vi "MoveVelocity.vi"(0 "reinitialize? (F)":bool, 1 "PID gains":T1={"proportional gain (Kc)"=0.6, "integral time (Ti, min)"=0.001, "derivative time (Td, min)"=0.0002}, 2 "output range":cluster{"output high":dbl, "output low":dbl}={"output high"=100.0, "output low"=-100.0}, 7 "EncRst":bool, 9 "OBJ":dbl[](array[numeric]), 11 "error in (no error)":errorcluster, 12 "dt (s)":dbl=0.010000000000000002 format="%#_13g") -> (6 "power":dbl[](array[numeric]), 8 "®t­È":dbl[](array[numeric]), 10 "Enc":dbl[](array[numeric]), 15 "error out":errorcluster)   [LabVIEW 2019]
uses:
  <vilib>/addons/control/pid/pid.llb/PID (DBL).vi
  <vilib>/addons/control/pid/NI_PID_pid.lvlib
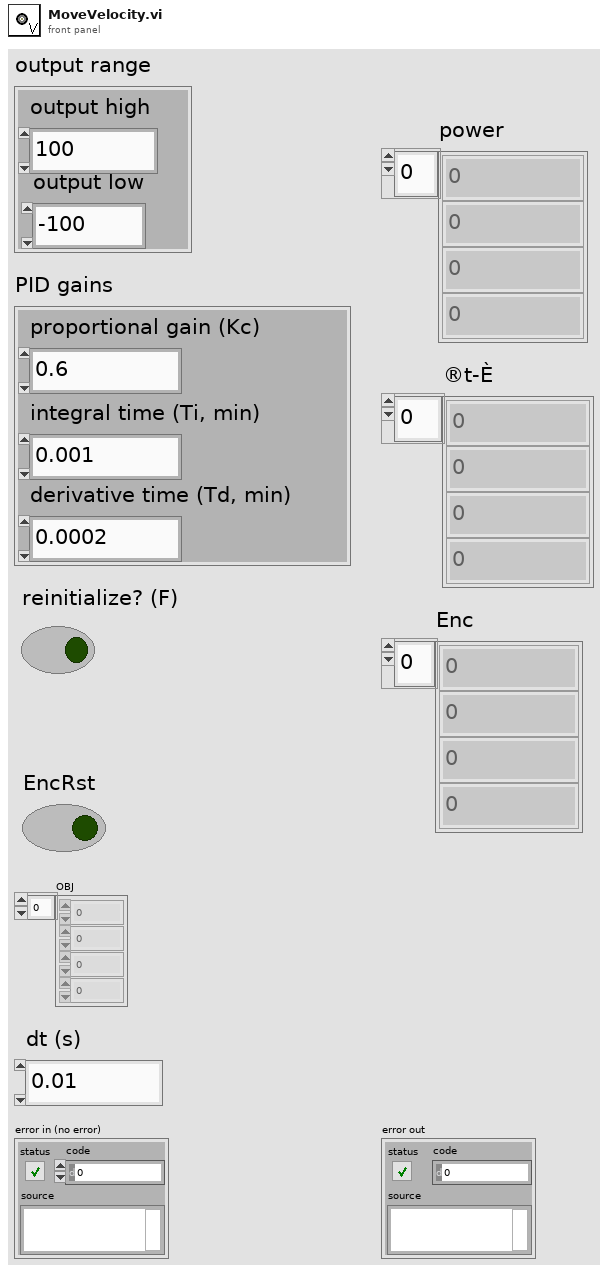
[diagram p1: front panel]
types:
  T1 = cluster{"proportional gain (Kc)":dbl, "integral time (Ti, min)":dbl, "derivative time (Td, min)":dbl}
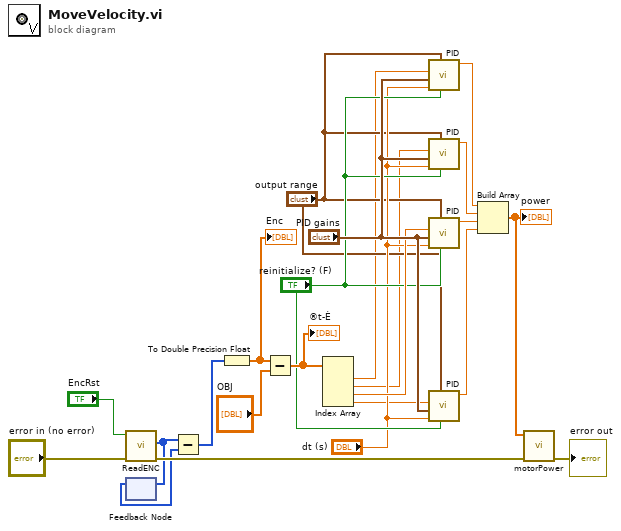
[diagram p0: block diagram]
diagram:
  n1 = call "ReadENC.vi"("error in (no error)"="error in (no error)", "Reset"="EncRst") -> ("error out"=w6:errorcluster, "ENC"=w2:i32[])  [unwired: 8 in]
  n2 = feedback-in #1(w2) -> ()
  n3 = feedback #1() -> (w1:i32[])  [unwired: 1 in]
  n4 = Subtract(x=w2, y=w1) -> (x-y=w20:i32[])
  n5 = To Double Precision Float(number=w20) -> (double precision float=w22:dbl[])
  "Enc" <- w22
  n6 = Subtract(x=w22, y="OBJ") -> (x-y=w21:dbl[])
  "®t­È" <- w21
  n7 = Index Array(array=w21) -> (element #1=w3:dbl, element #2=w4:dbl, element #3=w12:dbl, element #4=w9:dbl)  [unwired: 4 in]
  n8 = call-poly <vilib>:"PID.vi"("reinitialize? (F)"="reinitialize? (F)", "output range"="output range", "dt (s)"="dt (s)", "PID gains"="PID gains", "process variable"=w3) -> ("output"=w15:dbl)  [unwired: 5 in, 1 out]
  n9 = call-poly <vilib>:"PID.vi"("reinitialize? (F)"="reinitialize? (F)", "output range"="output range", "dt (s)"="dt (s)", "PID gains"="PID gains", "process variable"=w4) -> ("output"=w14:dbl)  [unwired: 5 in, 1 out]
  n10 = call-poly <vilib>:"PID.vi"("reinitialize? (F)"="reinitialize? (F)", "output range"="output range", "dt (s)"="dt (s)", "PID gains"="PID gains", "process variable"=w12) -> ("output"=w16:dbl)  [unwired: 5 in, 1 out]
  n11 = call-poly <vilib>:"PID.vi"("reinitialize? (F)"="reinitialize? (F)", "output range"="output range", "dt (s)"="dt (s)", "PID gains"="PID gains", "process variable"=w9) -> ("output"=w17:dbl)  [unwired: 5 in, 1 out]
  n12 = Build Array(w15, w14, w16, w17) -> (w7:dbl[])
  "power" <- w7
  n13 = call "motorPower.vi"("error in (no error)"=w6, "DC_Pwr"=w7) -> ("error out"=→"error out":errorcluster)  [unwired: 9 in]
